vi "Test Setup Error Dummy.vi"(8 "error in (no error)":errorcluster, 11 "Setup Error Test Dummy in":refnum<class "Setup Error Test Dummy.lvclass">) -> (0 "error out":errorcluster, 3 "Setup Error Test Dummy out":refnum<class "Setup Error Test Dummy.lvclass">)   [LabVIEW 2020, in "Teardown Error Test Dummy.lvclass"]
uses:
  Teardown Error Test Dummy.lvclass
  Teardown Error Test Dummy.lvclass/Teardown Error Test Dummy.ctl
  Core/LUnit Test Case/LUnit Test Case.lvclass
  Setup Error Test Dummy.lvclass
  C:/git/astemes-lunit/source/Core/LUnit Test Case/LUnit Test Case.lvclass
  C:/git/astemes-lunit/source/Core/Runnable/Runnable.lvclass
  C:/git/astemes-lunit/source/Tests/Error Checking Test/Dummys/Setup Error Test Dummy.lvclass
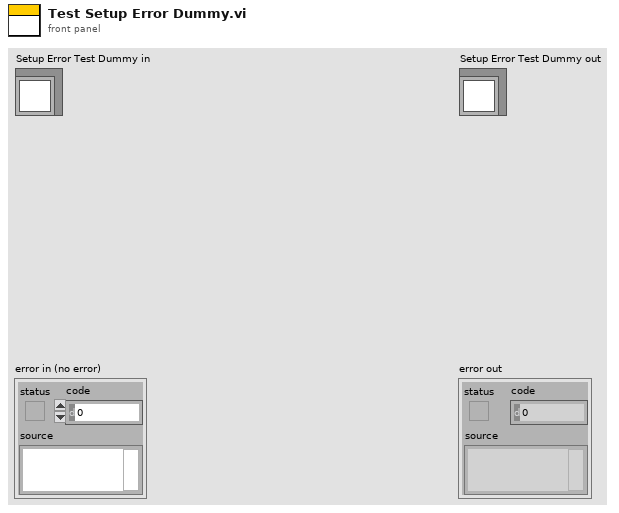
[diagram p1: front panel]
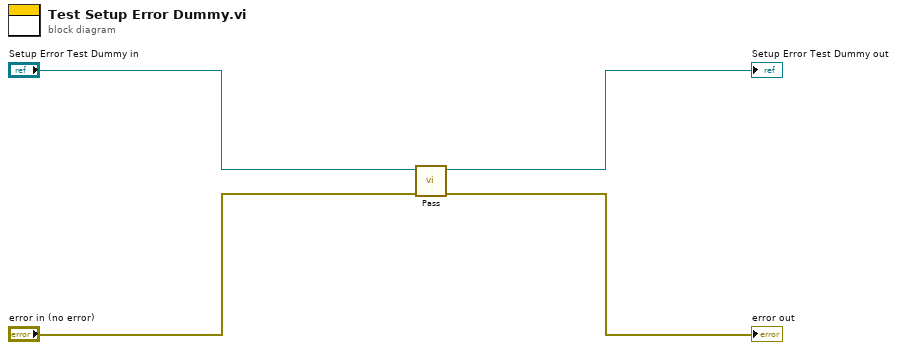
[diagram p0: block diagram]
diagram:
  n1 = call "Pass.vi"("error in (no error)"="error in (no error)", "LUnit Test Case In"="Setup Error Test Dummy in") -> ("error out"=→"error out":errorcluster, "LUnit Test Case Out"=→"Setup Error Test Dummy out":refnum<class "Setup Error Test Dummy.lvclass">)  [unwired: 8 in]
